vi "ATSh_SetRecordSize.vi"(9 "Length":u32, 10 "Presize":u32=1, 11 "HandleIn":u32) -> (0 "Return Code":u32, 3 "HandleOut":u32)   [LabVIEW 2015]
doc: "_____AlazarTech, Scope_____\n\nConfigure the record size information"
uses:
  ATSApi.dll
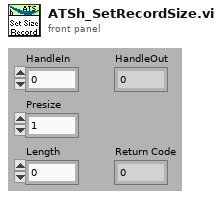
[diagram p1: front panel]
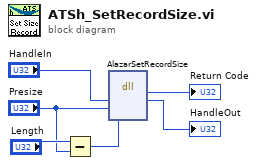
[diagram p0: block diagram]
diagram:
  n1 = Subtract(x="Length", y="Presize") -> (x-y=w1:u32)
  n2 = dll-call lib="C:/IntensityOCT/trunk/ATSApi.dll" fn="AlazarSetRecordSize"("h"="HandleIn", "Presize"="Presize", "Postsize"=w1) -> (→"Return Code":u32, "h"=→"HandleOut":u32)  [unwired: 5 in, 2 out]
